vi "REWORK_recolor_statuses.vi"(6 "Recolor? (T)":bool=TRUE, 8 "error_in":errorcluster, 10 "record_statuses":T1[](array[typedef]), 11 "listbox_ref":refnum<vi>) -> (0 "error_out":errorcluster)   [LabVIEW 2019]
uses:
  REWORK_gear_statuses.ctl
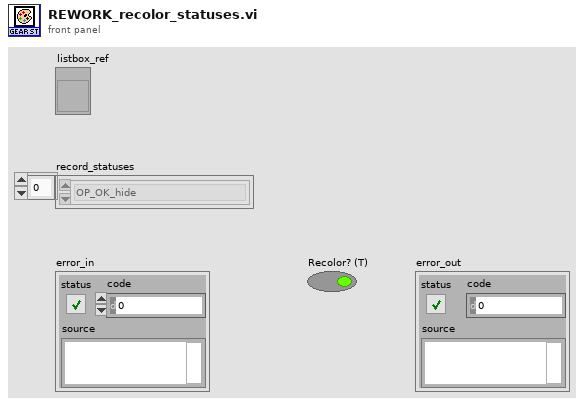
[diagram p1: front panel]
types:
  T1 = typedef "REWORK_gear_statuses.ctl" = enum16{"OP_OK_hide", "OP_OK_show", "OP_NOK_hide", "OP_NOK_show", "OP_interrupted_hide", "OP_interrupted_show", "OP_in_operation_hide", "OP_in_operation_show", "OP_unexpected_hide", "OP_unexpected_show", "RE_REAL_OK", "RE_REAL_NOK", "RE_STRING", "RE_sub_header", "RE_no_data", "RE_unexpected", "BA_sub_header", "BA_data", "BA_no_data"}
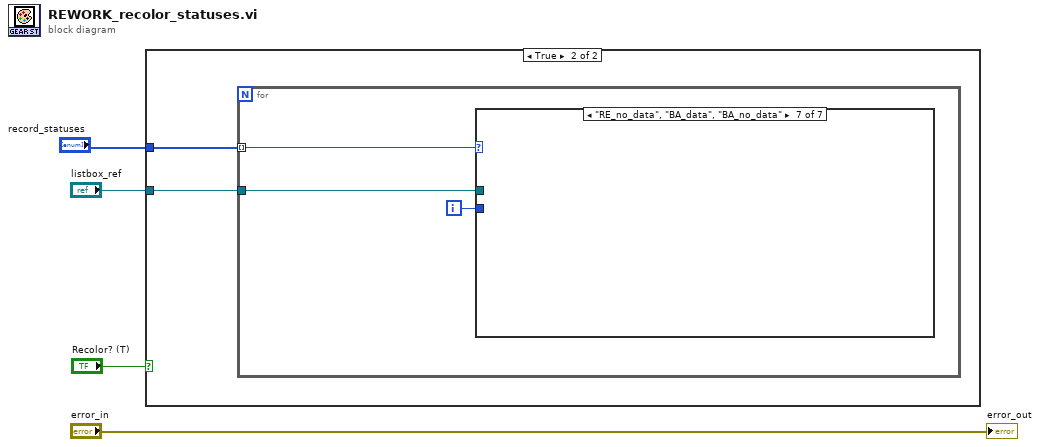
[diagram p0: block diagram]
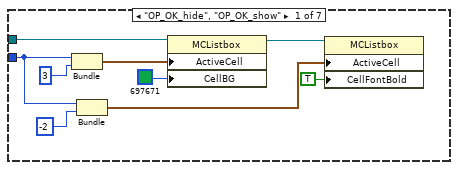
[diagram p3: hidden frame]
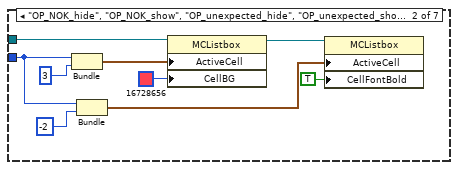
[diagram p4: hidden frame]
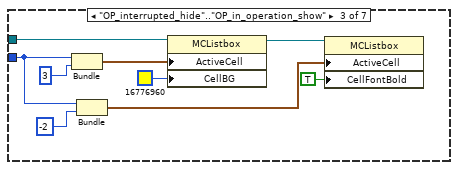
[diagram p5: hidden frame]
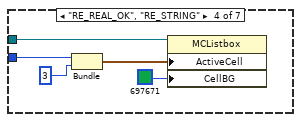
[diagram p6: hidden frame]
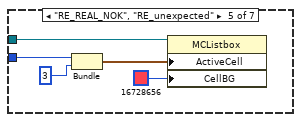
[diagram p7: hidden frame]
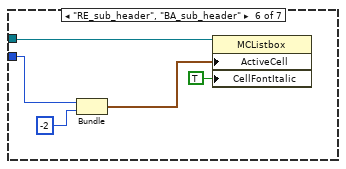
[diagram p8: hidden frame]
diagram:
  n1 = case shown="True" "Recolor? (T)" {
    tunnel: "record_statuses" -> [_ w5]
    tunnel: "listbox_ref" -> [_ w6]
    frame False {
    }
    frame True {
      n2 = for {
        tunnel: w6 -> [w9]
        tunnel: w5 -> [w8] mode=indexing
        i -> [w7]
        n3 = case shown="\"RE_no_data\", \"BA_data\", \"BA_no_data\"" w8 {
          tunnel: w9 -> [w16 w25 w34 w39 w44 w47 _]
          tunnel: w7 -> [w15 w24 w33 w38 w43 w51 _]
          frame "OP_OK_hide", "OP_OK_show" {
            n4 = Bundle(w15, 3) -> (w17:cluster{i32, i32})  [unwired: 1 in]
            n5 = Bundle(w15, -2) -> (w12:cluster{i32, i32})  [unwired: 1 in]
            n6 = property on="Property Node" class="MCListbox"(reference=w16, "ActiveCell"=w17, "CellBG"=u32 697671) -> (reference out=w13:refnum<vi>)  [unwired: 1 in, 1 out]
            n7 = property on="Property Node" class="MCListbox"(reference=w13, "ActiveCell"=w12, "CellFontBold"=TRUE ("Active Cell:Cell Font:Bold")) -> ()  [unwired: 1 in, 2 out]
          }
          frame "OP_NOK_hide", "OP_NOK_show", "OP_unexpected_hide", "OP_unexpected_show" {
            n8 = Bundle(w24, 3) -> (w26:cluster{i32, i32})  [unwired: 1 in]
            n9 = Bundle(w24, -2) -> (w21:cluster{i32, i32})  [unwired: 1 in]
            n10 = property on="Property Node" class="MCListbox"(reference=w25, "ActiveCell"=w26, "CellBG"=u32 16728656) -> (reference out=w22:refnum<vi>)  [unwired: 1 in, 1 out]
            n11 = property on="Property Node" class="MCListbox"(reference=w22, "ActiveCell"=w21, "CellFontBold"=TRUE ("Active Cell:Cell Font:Bold")) -> ()  [unwired: 1 in, 2 out]
          }
          frame "OP_interrupted_hide".."OP_in_operation_show" {
            n12 = Bundle(w33, 3) -> (w35:cluster{i32, i32})  [unwired: 1 in]
            n13 = Bundle(w33, -2) -> (w30:cluster{i32, i32})  [unwired: 1 in]
            n14 = property on="Property Node" class="MCListbox"(reference=w34, "ActiveCell"=w35, "CellBG"=u32 16776960) -> (reference out=w31:refnum<vi>)  [unwired: 1 in, 1 out]
            n15 = property on="Property Node" class="MCListbox"(reference=w31, "ActiveCell"=w30, "CellFontBold"=TRUE ("Active Cell:Cell Font:Bold")) -> ()  [unwired: 1 in, 2 out]
          }
          frame "RE_REAL_OK", "RE_STRING" {
            n16 = Bundle(w38, 3) -> (w40:cluster{i32, i32})  [unwired: 1 in]
            n17 = property on="Property Node" class="MCListbox"(reference=w39, "ActiveCell"=w40, "CellBG"=u32 697671) -> ()  [unwired: 1 in, 2 out]
          }
          frame "RE_REAL_NOK", "RE_unexpected" {
            n18 = Bundle(w43, 3) -> (w45:cluster{i32, i32})  [unwired: 1 in]
            n19 = property on="Property Node" class="MCListbox"(reference=w44, "ActiveCell"=w45, "CellBG"=u32 16728656) -> ()  [unwired: 1 in, 2 out]
          }
          frame "RE_sub_header", "BA_sub_header" {
            n20 = Bundle(w51, -2) -> (w49:cluster{i32, i32})  [unwired: 1 in]
            n21 = property on="Property Node" class="MCListbox"(reference=w47, "ActiveCell"=w49, "CellFontItalic"=TRUE ("Active Cell:Cell Font:Bold")) -> ()  [unwired: 1 in, 2 out]
          }
          frame "RE_no_data", "BA_data", "BA_no_data" {
          }
        }
      }
    }
  }
  "error_out" <- "error_in"
